vi "Benchmark_TCP Connection.vi"() -> ()   [LabVIEW 2013]
uses:
  source/Server/Connection/TCPConnection.lvclass
  source/MQTT_Base/MQTT_Base.lvclass
panel:
  in  "with Process":bool
  out "error out":errorcluster
  out "Waveform Chart":cluster{"elapsed (s)":dbl, "elapsed (s)":dbl}(graph)
  in  "stop":bool
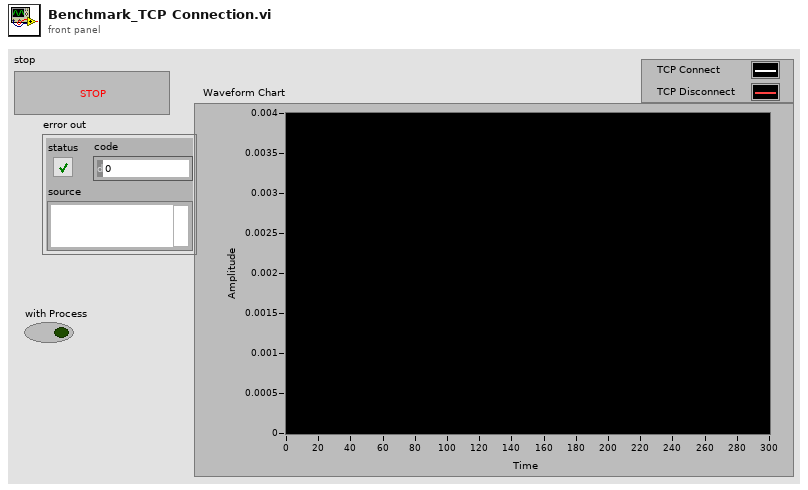
[diagram p1: front panel]
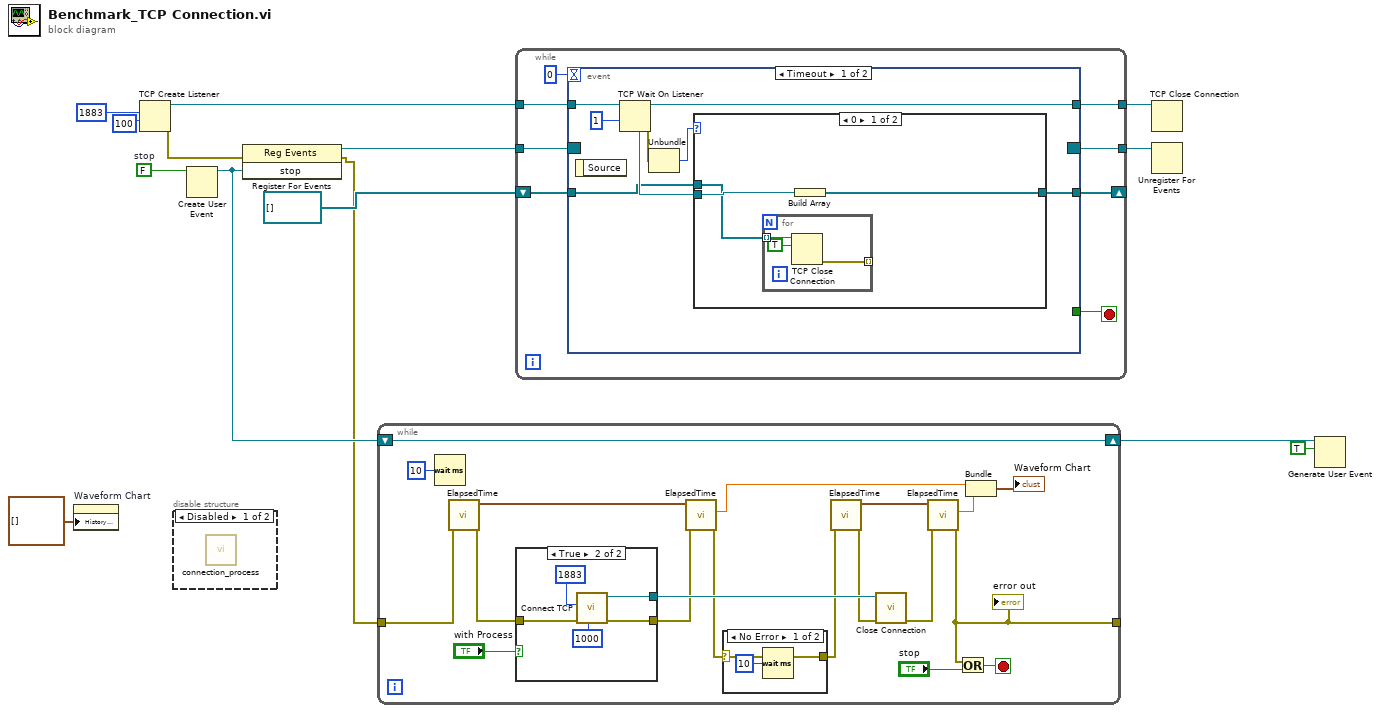
[diagram p0: block diagram]
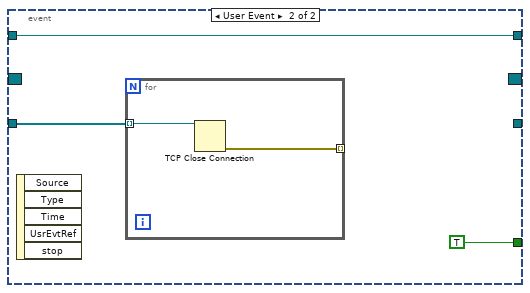
[diagram p3: hidden frame]
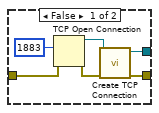
[diagram p4: hidden frame]
diagram:
  w13 = FALSE  # stop
  n1 = property on="Waveform Chart" class="WFChart (strict)"("History Data"=cluster{"elapsed (s)":dbl, "elapsed (s)":dbl}[] []) -> ()  [unwired: 2 in, 2 out]
  n2 = TCP Create Listener(9:100, 10:u16 1883 ("port")) -> (0:w1:errorcluster, 3:w5:refnum<k5>)  [unwired: 3 in, 1 out]
  n3 = disable-structure shown="Disabled" {
    frame Disabled {
      n4 = call "connection_process.vi"() -> ()  [unwired: 12 in]
    }
    frame Enabled {
    }
  }
  n5 = Create User Event(user event datatype=w13) -> (user event=w10:refnum<user-event>)  [unwired: 1 in, 1 out]
  n6 = register-events(error in=w1, w10) -> (reference out=w9:refnum<event-registration>, error out=w2:errorcluster)  [unwired: 1 in]
  n7 = while {
    tunnel: w2 -> [w32]
    tunnel: [w27] -> _
    shift-right: [w20] -> w12
    shift-left: w10 -> [w20]
    stop <- w26 stop-if-true
    n8 = Wait (ms)(milliseconds to wait=u32 10) -> ()  [unwired: 1 out]
    n9 = call "ElapsedTime.vi"("error in"=w32) -> ("error out"=w31:errorcluster, "current time"=w28:timestamp)  [unwired: 8 in, 1 out]
    n10 = case shown="True" "with Process" {
      tunnel: [w38 w44] -> w33
      tunnel: w31 -> [w35 w43]
      tunnel: [w39 w42] -> w30
      frame False {
        n11 = TCP Open Connection(remote port or service name=u16 1883, error in (no error)=w35) -> (connection ID=w37:refnum<k5>, error out=w34:errorcluster)  [unwired: 3 in]
        n12 = call "Create TCP Connection.vi"("error in (no error)"=w34, "connection ID"=w37) -> ("error out"=w39:errorcluster, "TCPConnection out"=w38:refnum<class "TCPConnection.lvclass">)  [unwired: 8 in]
      }
      frame True {
        n13 = call "Connect TCP.vi"("timeout (100ms)"=1000, "error in (no error)"=w43, "remote port (80)"=u16 1883) -> ("error out"=w42:errorcluster, "TCPConnection out"=w44:refnum<class "TCPConnection.lvclass">)  [unwired: 7 in]
      }
    }
    n14 = call "ElapsedTime.vi"("error in"=w30, "compare time"=w28) -> ("error out"=w17:errorcluster, "elapsed (s)"=w24:dbl)  [unwired: 7 in, 1 out]
    n15 = case shown="No Error" w17 {
      selector: w17 -> [w45 w47]
      tunnel: [w45 w47] -> w16
      frame No Error {
        n16 = Wait (ms)(milliseconds to wait=u32 10) -> ()  [unwired: 1 out]
      }
      frame Error {
      }
    }
    n17 = call "ElapsedTime.vi"("error in"=w16) -> ("error out"=w19:errorcluster, "current time"=w18:timestamp)  [unwired: 8 in, 1 out]
    n18 = call-dynamic "Close Connection.vi"("error in (no error)"=w19, "TCPConnection in"=w33) -> ("error out"=w29:errorcluster)  [unwired: 8 in, 1 out]
    n19 = call "ElapsedTime.vi"("error in"=w29, "compare time"=w18) -> ("error out"=w27:errorcluster, "elapsed (s)"=w23:dbl)  [unwired: 7 in, 1 out]
    "error out" <- w27
    n20 = Or(x=w27, y="stop") -> (x .or. y?=w26:bool)
    n21 = Bundle("elapsed (s)"=w24, "elapsed (s)"=w23) -> (→"Waveform Chart":cluster{"elapsed (s)":dbl, "elapsed (s)":dbl})  [unwired: 1 in]
  }
  n22 = while {
    tunnel: w9 -> [w55]
    tunnel: [w54] -> w8
    tunnel: w5 -> [w52]
    tunnel: [w50] -> w4
    shift-right: [w49] -> _
    shift-left: refnum<k5>[] [] -> [w48]
    stop <- w51 stop-if-true
    n23 = event shown="[0] Timeout" {
      selector: w55 -> [_ _]
      dyn-events: [_ _] -> w54
      timeout: 0 -> [_ _]
      tunnel: w52 -> [w62 w72]
      tunnel: [_ TRUE] -> w51
      tunnel: [w60 w72] -> w50
      tunnel: [w59 _] -> w49
      tunnel: w48 -> [w58 w71]
      event Timeout {
        n24 = event-data() -> ()  [unwired: 1 in, 1 out]
        n25 = TCP Wait On Listener(9:1, 11:w62) -> (0:w57:errorcluster, 3:w60:refnum<k5>, 4:w61:refnum<k5>)  [unwired: 2 in, 2 out]
        n26 = Unbundle(w57) -> ("code"=w56:i32)  [unwired: 2 out]
        n27 = case shown="0" w56 {
          tunnel: w61 -> [w65 _]
          tunnel: [w66 w70] -> w59
          tunnel: w58 -> [w64 w70]
          frame 0 {
            n28 = for {
              tunnel: w64 -> [w69] mode=indexing
              tunnel: [w68] -> _ mode=indexing
              n29 = TCP Close Connection(connection ID=w69, abort (F)=TRUE) -> (error out=w68:errorcluster)  [unwired: 1 in, 1 out]
            }
            n30 = Build Array(w65) -> (w66:refnum<k5>[])
          }
          frame Default {
          }
        }
      }
      event User Event {
        n31 = event-data() -> ()  [unwired: 1 in, 5 out]
        n32 = for {
          tunnel: w71 -> [w75] mode=indexing
          tunnel: [w74] -> _ mode=indexing
          n33 = TCP Close Connection(connection ID=w75) -> (error out=w74:errorcluster)  [unwired: 2 in, 1 out]
        }
      }
    }
  }
  n34 = TCP Close Connection(connection ID=w4) -> ()  [unwired: 2 in, 2 out]
  n35 = Unregister For Events(event registration refnum=w8) -> ()  [unwired: 1 in, 1 out]
  n36 = Generate User Event(user event=w12, event data cluster=TRUE ("event data")) -> ()  [unwired: 2 in, 2 out]
